vi "Get Current Temperature.vi"(8 "error in (no error)":errorcluster, 11 "Cooler in":refnum<class "Cooler.lvclass">) -> (0 "error out":errorcluster, 2 "Level":dbl)   [LabVIEW 2018, in "Cooler.lvlib" / "Cooler.lvclass"]
doc: "Read the current temperature from sensors or simulated hardware."
uses:
  Cooler.lvclass
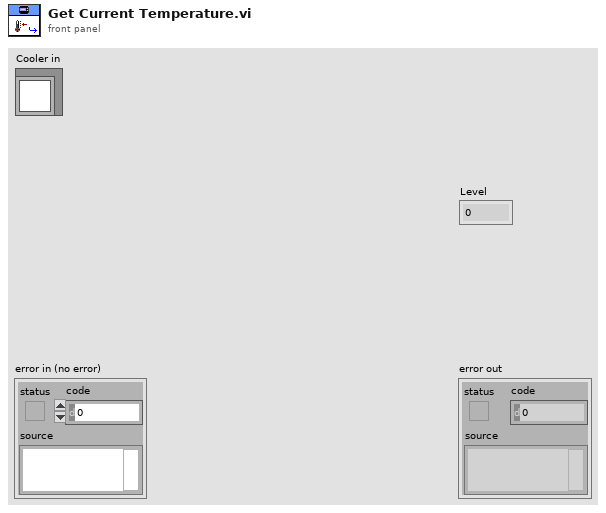
[diagram p1: front panel]
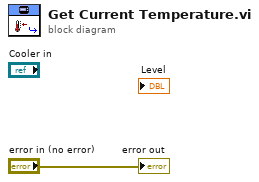
[diagram p0: block diagram]
diagram:
  "error out" <- "error in (no error)"
